vi "Add Tree Nodes.vi"(7 "Root path":string, 8 "Event Types":T1[](array[typedef]), 9 "map ref in":map{string, refnum<vi>}(c390), 10 "DQMH Lib In":refnum<vi>, 11 "Tree Map in":T2) -> (1 "map ref out":map{string, refnum<vi>}(c390), 3 "Tree Map out":T2)   [LabVIEW 2020, in "Dashboard.lvlib"]
uses:
  Dashboard.lvlib
  <vilib>/National Instruments/Tree Map/Tree Map Data.ctl
  Event types--enum.ctl
  <vilib>/Delacor/Delacor QMH/Libraries/Scripting API/DQMH_Scripting API.lvlib
  <vilib>/National Instruments/Tree Map/Tree Map.lvlib
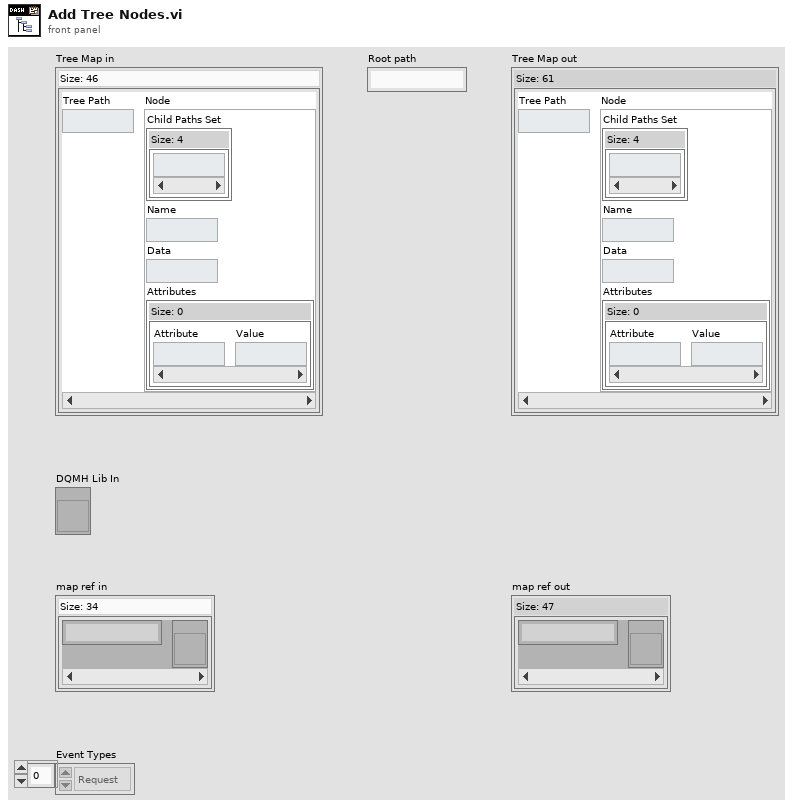
[diagram p1: front panel]
types:
  T1 = typedef "Dashboard.lvlib/Event types--enum.ctl" = enum16{"Request", "Request and Wait for Reply", "Broadcast"}
  T2 = typedef "Tree Map.lvlib/Tree Map Data.ctl" = map{string, cluster{"Child Paths Set":set{string}, "Name":string, "Data":string, "Attributes":map{string, string}}}
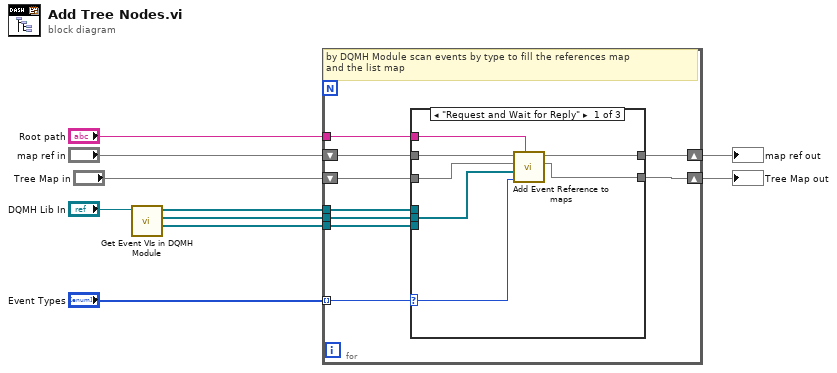
[diagram p0: block diagram]
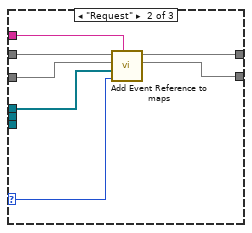
[diagram p2: hidden frame]
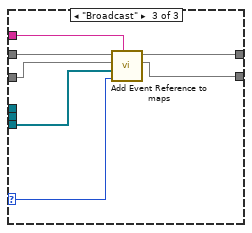
[diagram p3: hidden frame]
diagram:
  n1 = call <vilib>:"Get Event VIs in DQMH Module.vi"("DQMH Module"="DQMH Lib In") -> ("Broadcast Event VIs"=w1:refnum<vi>[], "Request and Wait for Reply Event VIs"=w2:refnum<vi>[], "Request Event VIs"=w3:refnum<vi>[])  [unwired: 7 in, 1 out]
  n2 = for {
    tunnel: "Root path" -> [w12]
    tunnel: "Event Types" -> [w13] mode=indexing
    shift-right: [w19] -> w10
    shift-left: "map ref in" -> [w18]
    shift-right: [w17] -> w7
    shift-left: "Tree Map in" -> [w11]
    tunnel: w3 -> [w16]
    tunnel: w2 -> [w15]
    tunnel: w1 -> [w14]
    # "by DQMH Module scan events by type to fill the references map\nand the list map"
    n3 = case shown="\"Request and Wait for Reply\"" w13 {
      selector: w13 -> [w21 w29 w36]
      tunnel: [w26 w33 w40] -> w19
      tunnel: w18 -> [w25 w32 w39]
      tunnel: [w24 w31 w38] -> w17
      tunnel: w16 -> [_ w27 _]
      tunnel: w15 -> [w22 _ _]
      tunnel: w14 -> [_ _ w35]
      tunnel: w12 -> [w20 w28 w34]
      tunnel: w11 -> [w23 w30 w37]
      frame "Request and Wait for Reply" {
        n4 = call "Add Event Reference to maps.vi"("New Node Path"=w20, "Event type"=w21, "Event VIs"=w22, "Tree Map in"=w23, "map ref in"=w25) -> ("Tree Map out"=w24:T2, "map ref out"=w26:map{string, refnum<vi>})  [unwired: 5 in]
      }
      frame "Request" {
        n5 = call "Add Event Reference to maps.vi"("New Node Path"=w28, "Event type"=w29, "Event VIs"=w27, "Tree Map in"=w30, "map ref in"=w32) -> ("Tree Map out"=w31:T2, "map ref out"=w33:map{string, refnum<vi>})  [unwired: 5 in]
      }
      frame "Broadcast" {
        n6 = call "Add Event Reference to maps.vi"("New Node Path"=w34, "Event type"=w36, "Event VIs"=w35, "Tree Map in"=w37, "map ref in"=w39) -> ("Tree Map out"=w38:T2, "map ref out"=w40:map{string, refnum<vi>})  [unwired: 5 in]
      }
    }
  }
  "map ref out" <- w10
  "Tree Map out" <- w7
